vi "Read Master.vi"(8 "error in":errorcluster, 10 "connection ID":refnum<k16>, 11 "TeleOp Data in":T1) -> (0 "error out":errorcluster, 3 "TeleOp Data out":T1)   [LabVIEW 2018]
uses:
  TypeDefs/Teleop Data Cluster.ctl
  TypeDefs/Input Read States.ctl
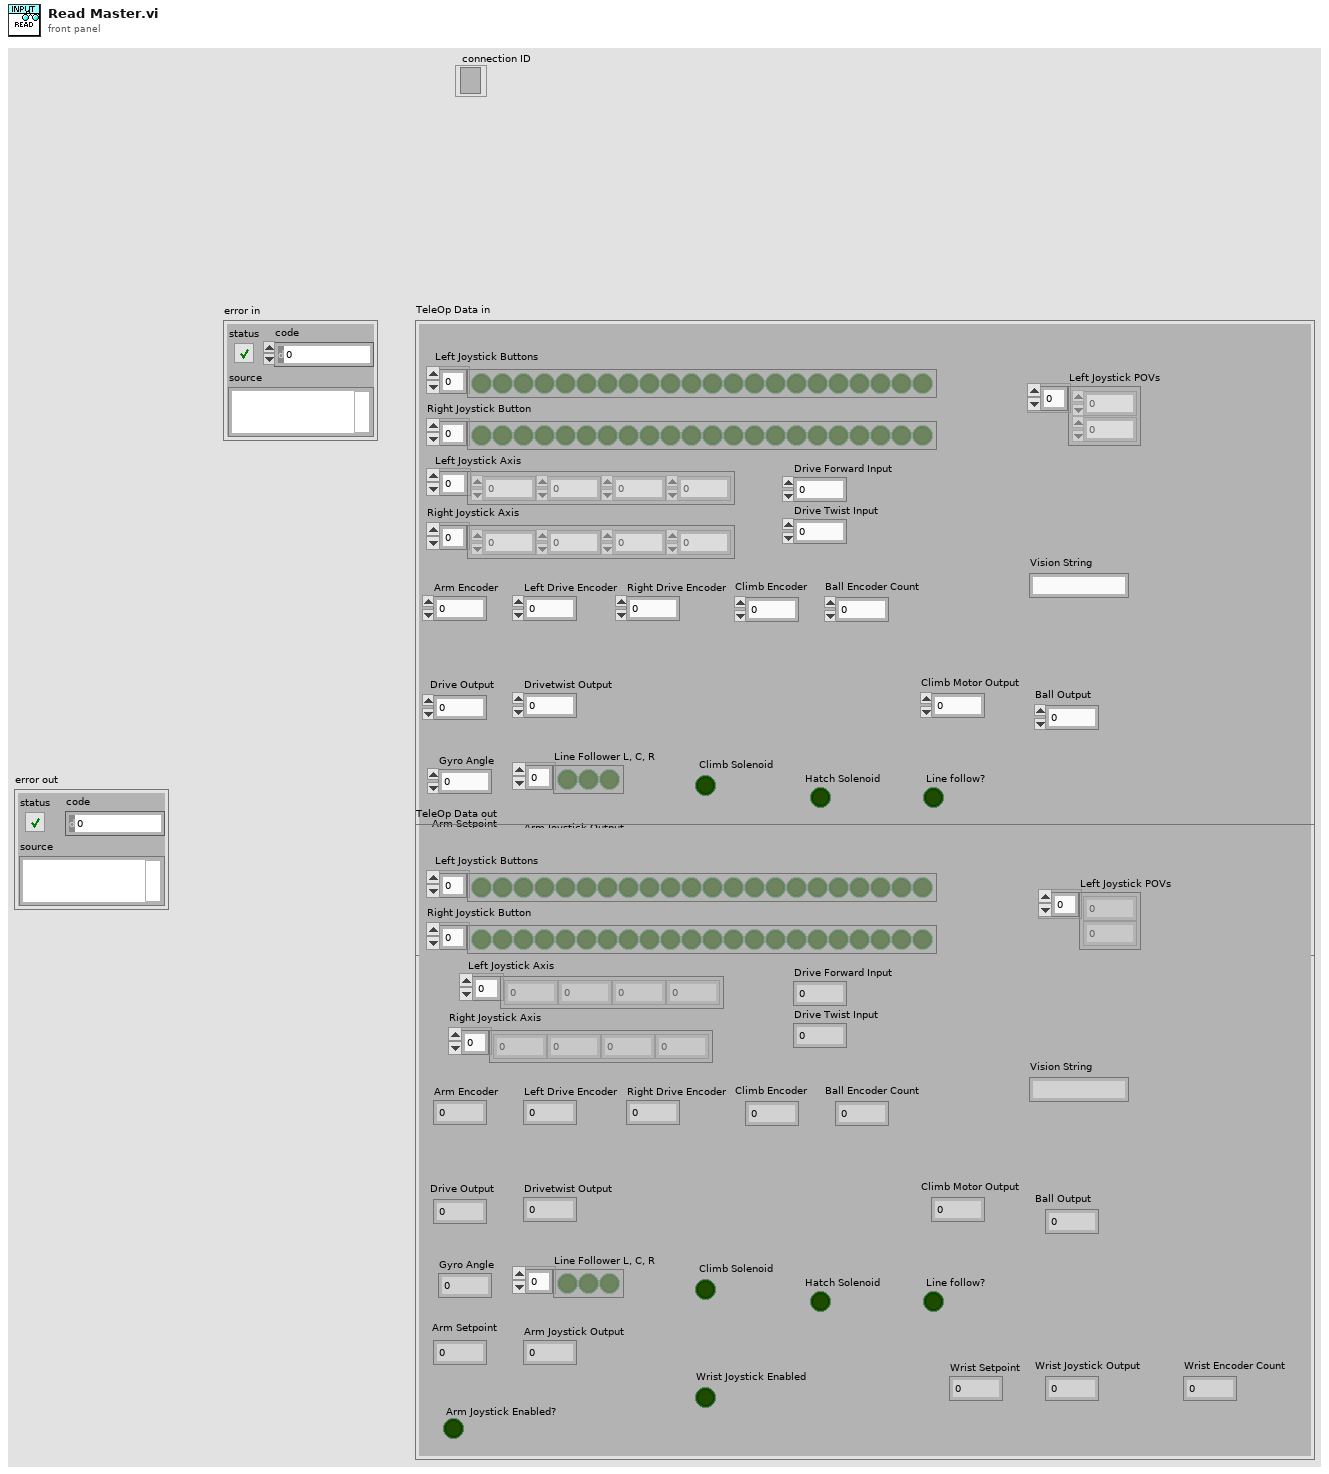
[diagram p1: front panel]
types:
  T1 = typedef "Teleop Data Cluster.ctl" = cluster{"Drive Forward Input ":dbl, "Drive Twist Input":dbl, "Drive Output":dbl, "Drivetwist Output":dbl, "Left Joystick Buttons":bool[], "Left Joystick Axis":dbl[], "Right Joystick Axis":dbl[], "Right Joystick Button":bool[], "Arm Encoder":dbl, "Left Drive Encoder":dbl, "Right Drive Encoder":dbl, "Gyro Angle ":dbl, "Arm Joystick Output  ":dbl, "Line Follower L, C, R ":bool[], "Line follow?":bool, " Climb Solenoid":bool, "Wrist Encoder Count":dbl, "Wrist Joystick Output":dbl, "Ball Encoder Count":dbl, "Ball Output":dbl, "Climb Encoder":dbl, "Climb Motor Output":dbl, " Hatch Solenoid":bool, "Arm Setpoint ":dbl, "Wrist Setpoint ":dbl, "Arm Joystick Enabled?":bool, "Wrist Joystick Enabled":bool, "Vision String":string, "Left Joystick POVs":i16[]}
  T2 = typedef "Input Read States.ctl" = enum16{"Read Joysticks", "Read Encoders", "Read Gyro", "Read Line Followers", "Read Complete"}
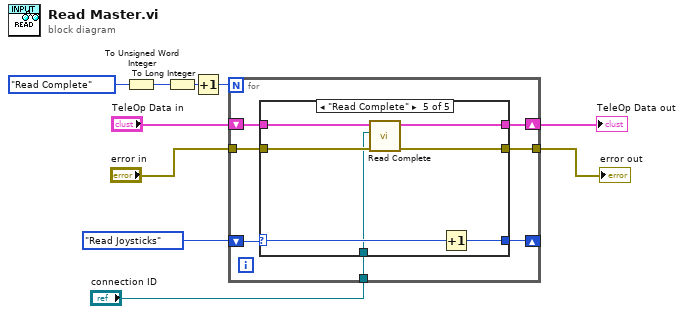
[diagram p0: block diagram]
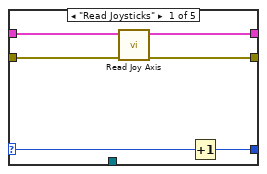
[diagram p2: hidden frame]
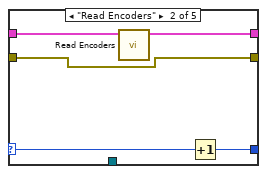
[diagram p3: hidden frame]
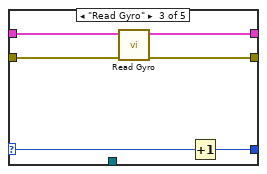
[diagram p4: hidden frame]
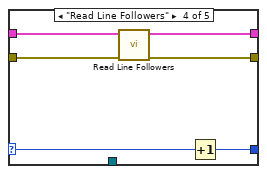
[diagram p5: hidden frame]
diagram:
  n1 = To Unsigned Word Integer(number=Input_Read_States."Read Complete" ("Enum")) -> (unsigned 16bit integer=w6:u16)
  n2 = To Long Integer(number=w6) -> (32bit integer=w5:i32)
  n3 = Increment(x=w5) -> (x+1=w1:i32)
  n4 = for {
    N: w1 -> [_]
    shift-right: [w15] -> w9
    shift-left: "TeleOp Data in" -> [w14]
    shift-right: [w16] -> _
    shift-left: Input_Read_States."Read Joysticks" ("Enum") -> [w17]
    tunnel: "error in" -> [w13]
    tunnel: [w12] -> w3
    tunnel: "connection ID" -> [w11]
    n5 = case shown="\"Read Complete\"" w17 {
      selector: w17 -> [w23 w28 w34 w40 w47]
      tunnel: [w22 w27 w33 w39 w46] -> w16
      tunnel: [w20 w25 w31 w37 w44] -> w15
      tunnel: w14 -> [w21 w26 w32 w38 w45]
      tunnel: w13 -> [w19 w24 w30 w36 w43]
      tunnel: [w18 w24 w29 w35 w42] -> w12
      tunnel: w11 -> [_ _ _ _ w41]
      frame "Read Joysticks" {
        n6 = call "Read Joy Axis.vi"("error in"=w19, "TeleOp Data Cluster in"=w21) -> ("error out"=w18:errorcluster, "TeleOp Data Cluster out"=w20:T1)  [unwired: 8 in]
        n7 = Increment(x=w23) -> (x+1=w22:T2)
      }
      frame "Read Encoders" {
        n8 = call "Read Encoders.vi"("TeleOp Data Cluster in"=w26) -> ("TeleOp Data Cluster out"=w25:T1)  [unwired: 9 in, 1 out]
        n9 = Increment(x=w28) -> (x+1=w27:T2)
      }
      frame "Read Gyro" {
        n10 = call "Read Gyro.vi"("error in"=w30, "TeleOp Data Cluster in"=w32) -> ("error out"=w29:errorcluster, "TeleOp Data Cluster out"=w31:T1)  [unwired: 8 in]
        n11 = Increment(x=w34) -> (x+1=w33:T2)
      }
      frame "Read Line Followers" {
        n12 = call "Read Line Followers.vi"("error in"=w36, "TeleOp Data Cluster in"=w38) -> ("error out"=w35:errorcluster, "Teleop Data Cluster out"=w37:T1)  [unwired: 8 in]
        n13 = Increment(x=w40) -> (x+1=w39:T2)
      }
      frame "Read Complete" {
        n14 = call "Read Complete.vi"("error in"=w43, "connection ID"=w41, "TeleOp Data Cluster in"=w45) -> ("error out"=w42:errorcluster, "TeleOp Data Cluster out"=w44:T1)  [unwired: 7 in]
        n15 = Increment(x=w47) -> (x+1=w46:T2)
      }
    }
  }
  "TeleOp Data out" <- w9
  "error out" <- w3
